vi "Calc Dist to ConstV.vi"(9 "V2 (fps)":dbl=10.0, 10 "Limits":T3={"Acceleration (fps^2)"=10.0, "Jerk (fps^3)"=100.0}, 11 "V1  (fps)":dbl) -> (1 "distances":T2, 2 "timings":T1, 3 "distance (ft)":dbl)   [LabVIEW 2025]
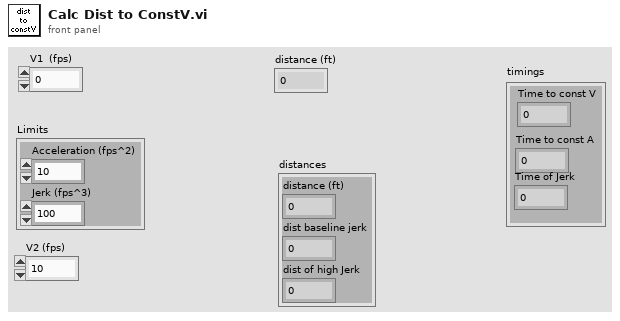
[diagram p1: front panel]
types:
  T1 = cluster{"Time to const V":dbl, "Time to const A":dbl, "Time of Jerk":dbl}
  T2 = cluster{"distance (ft)":dbl, "dist baseline jerk":dbl, "dist of high Jerk":dbl}
  T3 = cluster{"Acceleration (fps^2)":dbl, "Jerk (fps^3)":dbl}
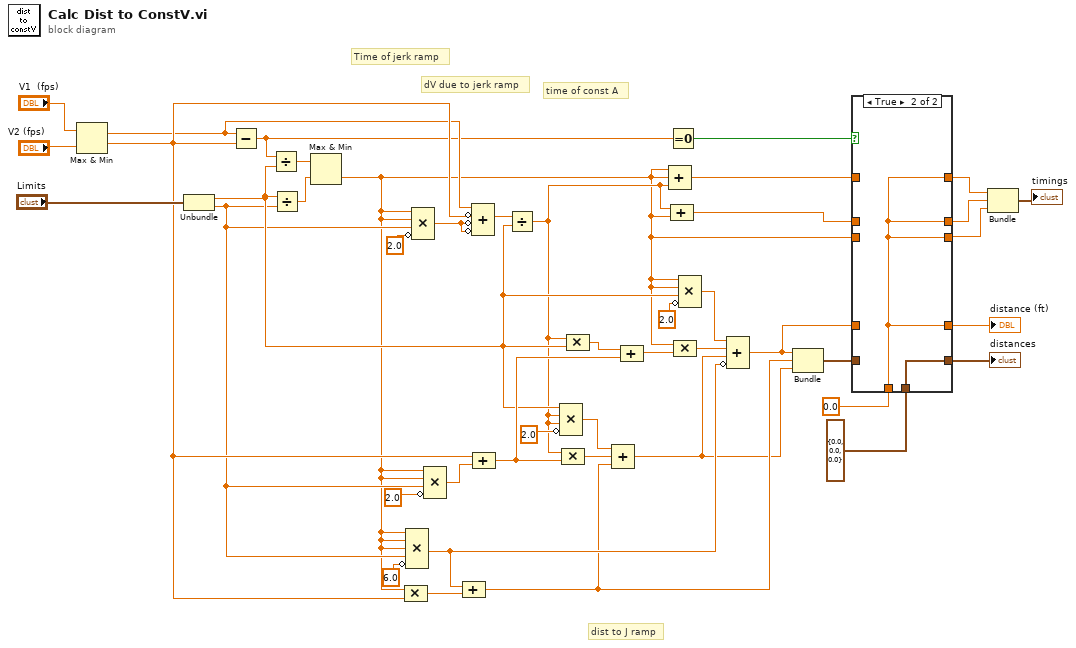
[diagram p0: block diagram]
diagram:
  # "dist to J ramp"
  # "time of const A"
  # "dV due to jerk ramp"
  # "Time of jerk ramp"
  n1 = Max & Min(x="V1  (fps)", y="V2 (fps)") -> (max(x,y)=w19:dbl, min(x,y)=w20:dbl)
  n2 = Unbundle("Limits") -> ("Acceleration (fps^2)"=w18:dbl, "Jerk (fps^3)"=w17:dbl)
  n3 = Subtract(x=w19, y=w20) -> (x-y=w16:dbl)
  n4 = Divide(x=w16, y=w18) -> (x/y=w26:dbl)
  n5 = Divide(x=w18, y=w17) -> (x/y=w25:dbl)
  n6 = Max & Min(x=w26, y=w25) -> (min(x,y)=w2:dbl)  [unwired: 1 out]
  n7 = Compound Arithmetic op=MULTIPLY(w2, w20) -> (w38:dbl)
  n8 = Compound Arithmetic op=MULTIPLY(w2, w2, w2, w17, invert 6.0) -> (w30:dbl)
  n9 = Compound Arithmetic op=MULTIPLY(w2, w2, w17, invert 2.0) -> (w39:dbl)
  n10 = Compound Arithmetic op=MULTIPLY(w2, w2, w17, invert 2.0) -> (w29:dbl)
  n11 = Compound Arithmetic op=ADD(w30, w38) -> (w24:dbl)
  n12 = Compound Arithmetic op=ADD(w19, invert w20, invert w39, invert w39) -> (w42:dbl)
  n13 = Compound Arithmetic op=ADD(w20, w29) -> (w33:dbl)
  n14 = Divide(x=w42, y=w18) -> (x/y=w4:dbl)
  n15 = Compound Arithmetic op=MULTIPLY(w18, w4, w4, invert 2.0) -> (w36:dbl)
  n16 = Compound Arithmetic op=MULTIPLY(w4, w33) -> (w37:dbl)
  n17 = Compound Arithmetic op=MULTIPLY(w4, w18) -> (w32:dbl)
  n18 = Compound Arithmetic op=ADD(w36, w37, w24) -> (w23:dbl)
  n19 = Compound Arithmetic op=ADD(w32, w33) -> (w31:dbl)
  n20 = Equal To 0?(x=w16) -> (x = 0?=w15:bool)
  n21 = Compound Arithmetic op=ADD(w2, w2, w4) -> (w14:dbl)
  n22 = Compound Arithmetic op=ADD(w4, w2) -> (w3:dbl)
  n23 = Compound Arithmetic op=MULTIPLY(w2, w31) -> (w35:dbl)
  n24 = Compound Arithmetic op=MULTIPLY(w2, w2, w18, invert 2.0) -> (w27:dbl)
  n25 = Compound Arithmetic op=ADD(w27, w35, w23, invert w30) -> (w13:dbl)
  n26 = Bundle(w13, w24, w23) -> (w12:cluster{dbl, dbl, dbl})  [unwired: 1 in]
  n27 = case shown="True" w15 {
    tunnel: w14 -> [w47 _]
    tunnel: w13 -> [w48 _]
    tunnel: w12 -> [w49 _]
    tunnel: [w49 w51] -> w11
    tunnel: [w48 w50] -> w10
    tunnel: [w47 w50] -> w7
    tunnel: cluster{dbl, dbl, dbl} {0.0, 0.0, 0.0} ("output cluster") -> [_ w51]
    tunnel: 0.0 -> [_ w50]
    tunnel: w3 -> [w46 _]
    tunnel: [w46 w50] -> w6
    tunnel: [w45 w50] -> w1
    tunnel: w2 -> [w45 _]
    frame False {
    }
    frame True {
    }
  }
  "distances" <- w11
  "distance (ft)" <- w10
  n28 = Bundle(w7, w6, w1) -> (→"timings":cluster{dbl, dbl, dbl})  [unwired: 1 in]
